vi "Create.vi"(8 "error in (no error)":errorcluster, 9 "ID":i32, 10 "Name":string, 11 "Motor in":refnum<class "Motor-Sieve2.lvclass">) -> (0 "error out":errorcluster, 3 "Motor out":refnum<class "Motor-Sieve2.lvclass">)   [LabVIEW 2013, in "PowderDeposition.lvlib" / "Motor-Sieve2.lvclass"]
uses:
  Motor-Sieve2.lvclass
  Units.ctl
  Action-settings.ctl
  Motor-GWInstek.lvclass/Motor-GWInstek.ctl
  Write Serial Configuration.vi
  Write Channel.vi
  Motor.lvclass
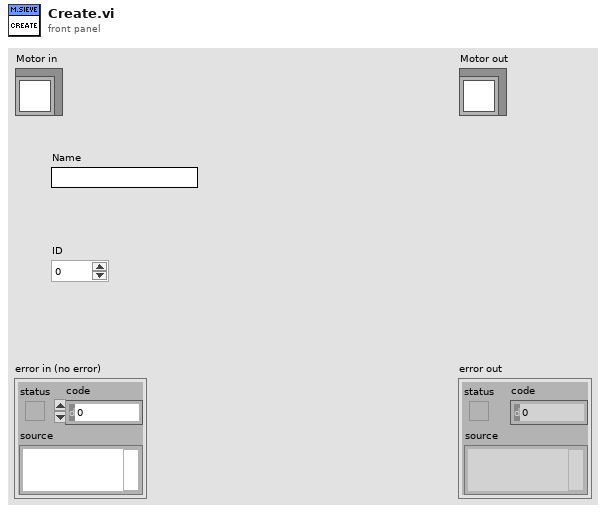
[diagram p1: front panel]
types:
  T1 = cluster{"Baud Rate":u32, "Parity":u16, "Data Bits":u16, "Stop Bits":u16, "Flow Control":u16}
  T2 = typedef "PowderDeposition.lvlib/Motor.lvclass/Action-settings.ctl" = cluster{"Speed":dbl, "Acceleration":dbl, "Direction":enum16{"Clockwise", "Counter-clockwise"}}
  T3 = typedef "PowderDeposition.lvlib/Motor.lvclass/Units.ctl" = enum16{"-", "mm", "µm", "tr", "V"}
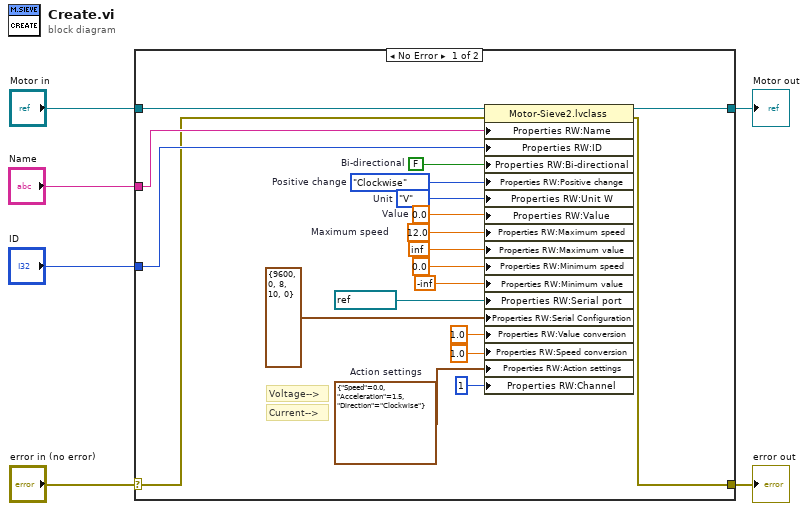
[diagram p0: block diagram]
diagram:
  n1 = case shown="No Error" "error in (no error)" {
    selector: "error in (no error)" -> [w13 w28]
    tunnel: [w14 w28] -> w5
    tunnel: [w15 w27] -> w3
    tunnel: "Motor in" -> [w26 w27]
    tunnel: "Name" -> [w25 _]
    tunnel: "ID" -> [w24 _]
    frame No Error {
      w11 = T2 {"Speed"=0.0, "Acceleration"=1.5, "Direction"=enum."Clockwise"}  # Action settings
      w19 = 12.0  # Maximum speed
      w20 = 0.0  # Value
      w21 = Units."V"  # Unit
      w22 = enum16{"Clockwise", "Counter-clockwise"}."Clockwise"  # Positive change
      w23 = FALSE  # Bi-directional
      # "Current-->"
      # "Voltage-->"
      n2 = property class="Motor-Sieve2.lvclass"(reference=w26, error in=w13, "Properties RW:Name"=w25, "Properties RW:ID"=w24, "Properties RW:Bi-directional"=w23, "Properties RW:Positive change"=w22, "Properties RW:Unit W"=w21, "Properties RW:Value"=w20, "Properties RW:Maximum speed"=w19, "Properties RW:Maximum value"=inf, "Properties RW:Minimum speed"=0.0 ("Minimum voltage"), "Properties RW:Minimum value"=-inf, "Properties RW:Serial port"=refnum<visa-resource-name> "COM6" ("Serial port"), "Properties RW:Serial Configuration"=T1 {"Baud Rate"=9600, "Parity"=0, "Data Bits"=8, "Stop Bits"=10, "Flow Control"=0} ("Serial Configuration"), "Properties RW:Value conversion"=1.0 ("Speed conversion"), "Properties RW:Speed conversion"=1.0 ("Value conversion"), "Properties RW:Action settings"=w11, "Properties RW:Channel"=1 ("Channel")) -> (reference out=w15:refnum<class "Motor-Sieve2.lvclass">, error out=w14:errorcluster)
    }
    frame Error {
    }
  }
  "error out" <- w5
  "Motor out" <- w3
